vi "Write.vi"(8 "error in (no error)":errorcluster, 10 "Data":dbl, 11 "RTFIFODouble in":refnum<class "CIFTag.lvclass">) -> (0 "error out":errorcluster, 1 "timed out?":bool, 3 "RTFIFODouble out":refnum<class "CIFTag.lvclass">)   [LabVIEW 2021, in "CIFTag.lvclass"]
uses:
  CIFTag.lvclass
  CIFTag.lvclass/CIFTag.ctl
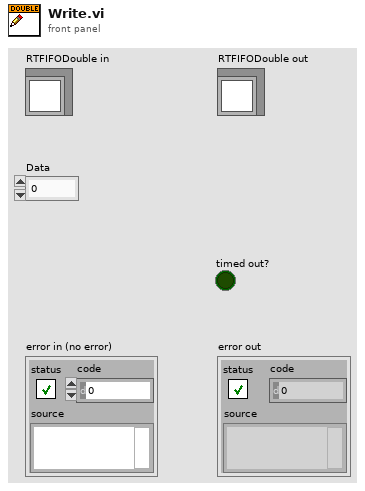
[diagram p1: front panel]
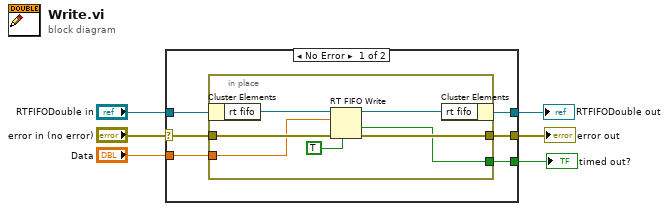
[diagram p0: block diagram]
diagram:
  n1 = case shown="No Error" "error in (no error)" {
    selector: "error in (no error)" -> [w10 w21]
    tunnel: [w9 w21] -> w5
    tunnel: [w11 w20] -> w3
    tunnel: "RTFIFODouble in" -> [w12 w20]
    tunnel: "Data" -> [w8 _]
    tunnel: [w7 _] -> w1
    frame No Error {
      n2 = in-place {
        in-place-border: w10 -> [w17]
        in-place-border: [w16] -> w9
        in-place-border: w8 -> [w15]
        in-place-border: [w13] -> w7
        n3 = in-place-cluster #1(w12) -> ("rt fifo"=w19:refnum<k33>)
        n4 = RT FIFO Write(0:w19, 1:w15, 3:w17, 5:TRUE ("overwrite on timeout (T)")) -> (8:w18:refnum<k33>, 10:w13:bool, 11:w16:errorcluster)  [unwired: 1 in, 1 out]
        n5 = in-place-cluster #1("rt fifo"=w18) -> (w11:refnum<class "CIFTag.lvclass">)
      }
    }
    frame Error {
    }
  }
  "error out" <- w5
  "RTFIFODouble out" <- w3
  "timed out?" <- w1
